vi "_io_viClear.vi"(6 "Block Logging (F)":bool, 8 "error in":errorcluster caption="error in (no error)", 11 "VISA resource name":refnum<visa-resource-name>) -> (0 "error out":errorcluster, 3 "VISA resource name out":refnum<visa-resource-name>)   [LabVIEW 2022 SP3, in "hmp4000_rsidr_core.lvlib"]
uses:
  hmp4000_rsidr_core.lvlib
  type_AdditionalFlag_Bits.ctl
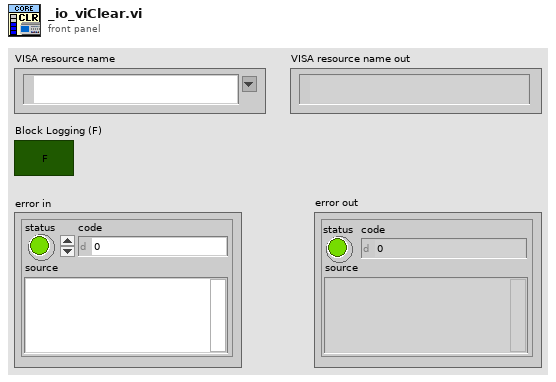
[diagram p1: front panel]
types:
  T1 = typedef "hmp4000_rsidr_core.lvlib/type_AdditionalFlag_Bits.ctl" = enum16{"Send LF after Bin Block", "Junk read with io_clear_buffers.vi", "io_clear_buffers: viClear()", "io_clear_buffers: viFlush()", "<NotUsed1>", "Allow Dbl & Int Bin/Ascii read", "*OPC? in check_instrument_error.vi", "<NotUsed2>", "Smart Enum Matching", "Less Strict RepCaps check", "AssureResponseEndWithLF"}
  T2 = typedef "hmp4000_rsidr_core.lvlib/type_Session_Data.ctl" = cluster{"IDN string":string, "Instrument FW":string, "Instr type":string, "Instr type for err. msg.":string, "Installed Options":string[], "Ignore Error Messages":string, "Logging params":variant, "OPC Timeout":i32, "VISA Timeout":i32, "STB Poll VISA Timeout":i32, "Additional Flags":i32, "Wait Before Read":i32, "Wait Before Write":i32, "Option String Flags":i32, "IO Segment Size":i64, "VISA Access Mode":T3, "Interface Type":T4, "OPC Wait Mode":T5, "Bin Float Number  Format":T6, "Bin Integer Number Format":T7, "Simulate":bool, "VXIcapable":bool, "Duplicate Session":bool, "Add LF to Write":bool, "Logging":bool, "Fast Sweep":bool, "Query Instrument Status":bool, "Check Range":bool, "Check Options":bool}
  T3 = typedef "hmp4000_rsidr_core.lvlib/type_VisaAccessMode.ctl" = u16
  T4 = typedef "hmp4000_rsidr_core.lvlib/type_InterfaceType.ctl" = enum16{"Unknown", "GPIB", "VXI", "GPIB_VXI", "ASRL", "PXI", "TCPIP", "USB", "SOCKET"}
  T5 = typedef "hmp4000_rsidr_core.lvlib/type_OPC_Wait_Mode.ctl" = enum16{"STBpolling", "STBpollingSlow", "STBpollingSuperSlow", "ServiceRequest", "OPCquery"}
  T6 = typedef "hmp4000_rsidr_core.lvlib/type_Binary_Float_Number_Format.ctl" = enum16{"Float_4_Bytes_Swapped", "Float_4_Bytes", "Double_8_Bytes_Swapped", "Double_8_Bytes"}
  T7 = typedef "hmp4000_rsidr_core.lvlib/type_Binary_Integer_Number_Format.ctl" = enum16{"Int32_4_Bytes_Swapped", "Int32_4 Bytes", "Int16_2_Bytes_Swapped", "Int16_2_Bytes"}
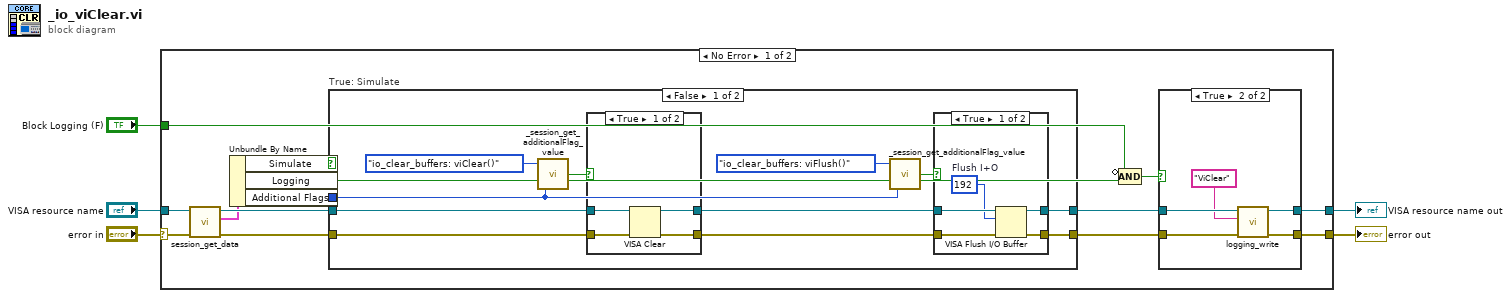
[diagram p0: block diagram]
diagram:
  n1 = case shown="No Error" "error in" {
    selector: "error in" -> [w19 w54]
    tunnel: [w13 w54] -> w1
    tunnel: "VISA resource name" -> [w18 w53]
    tunnel: [w10 w53] -> w2
    tunnel: "Block Logging (F)" -> [w6 _]
    frame No Error {
      n2 = call "session_get_data.vi"("error in"=w19, "VISA resource name"=w18) -> ("error out"=w17:errorcluster, "Session User Data out"=w15:T2, "VISA resource name out"=w16:refnum<visa-resource-name>)  [unwired: 6 in, 1 out]
      n3 = Unbundle By Name(w15) -> ("Simulate"=w14:bool, "Logging"=w9:bool, "Additional Flags"=w7:i32)
      n4 = case "True: Simulate" shown="False" w14 {
        tunnel: [w28 w52] -> w12
        tunnel: w17 -> [w37 w52]
        tunnel: w16 -> [w36 w51]
        tunnel: [w27 w51] -> w11
        tunnel: w7 -> [w29 _]
        frame False {
          n5 = call "_session_get_additionalFlag_value.vi"("AdditionalFlags value in"=w29, "AdditionalFlag bit"=type_AdditionalFlag_Bits."io_clear_buffers: viClear()") -> ("AdditionalFlag bit value out"=w33:bool)  [unwired: 3 in]
          n6 = case shown="True" w33 {
            tunnel: w37 -> [w48 w49]
            tunnel: w36 -> [w47 w50]
            tunnel: [w46 w49] -> w35
            tunnel: [w45 w50] -> w34
            frame True {
              n7 = VISA Clear(VISA resource name=w47, error in (no error)=w48) -> (VISA resource name out=w45:refnum<visa-resource-name>, error out=w46:errorcluster)
            }
            frame False {
            }
          }
          n8 = call "_session_get_additionalFlag_value.vi"("AdditionalFlags value in"=w29, "AdditionalFlag bit"=type_AdditionalFlag_Bits."io_clear_buffers: viFlush()") -> ("AdditionalFlag bit value out"=w30:bool)  [unwired: 3 in]
          n9 = case shown="True" w30 {
            tunnel: w35 -> [w42 w44]
            tunnel: w34 -> [w41 w43]
            tunnel: [w40 w44] -> w28
            tunnel: [w39 w43] -> w27
            frame True {
              w38 = u16 192  # Flush I+O
              n10 = VISA Flush I/O Buffer(VISA resource name=w41, mask (16)=w38, error in (no error)=w42) -> (VISA resource name out=w39:refnum<visa-resource-name>, error out=w40:errorcluster)
            }
            frame False {
            }
          }
        }
        frame True {
        }
      }
      n11 = Compound Arithmetic op=AND(invert w6, w9) -> (w8:bool)
      n12 = case shown="True" w8 {
        tunnel: w12 -> [w21 w26]
        tunnel: [w21 w24] -> w13
        tunnel: w11 -> [w20 w25]
        tunnel: [w20 w23] -> w10
        frame False {
        }
        frame True {
          n13 = call "logging_write.vi"("error in"=w26, "String to write"="ViClear", "VISA resource name"=w25) -> ("error out"=w24:errorcluster, "VISA resource name out"=w23:refnum<visa-resource-name>)  [unwired: 7 in]
        }
      }
    }
    frame Error {
    }
  }
  "VISA resource name out" <- w2
  "error out" <- w1
